vi "Curtin_convertrawData.vi"(0 "incoming data":waveform(dbl)[](array[waveform]), 1 "Ports":cluster{"mic":u8, "hammer":u8, "flip?":bool}={"mic"=1, "hammer"=2, "flip?"=FALSE}) -> (2 "Ordered":waveform(dbl)[](array[waveform]))   [LabVIEW 2022 SP3]
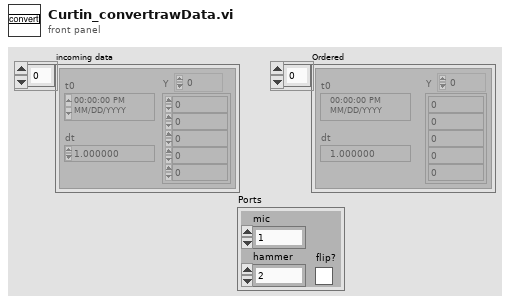
[diagram p1: front panel]
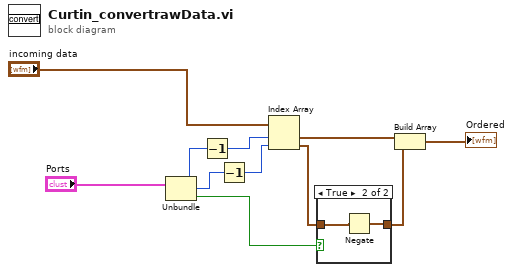
[diagram p0: block diagram]
diagram:
  n1 = Unbundle("Ports") -> ("mic"=w10:u8, "hammer"=w9:u8, "flip?"=w3:bool)
  n2 = Decrement(x=w10) -> (x-1=w2:u8)
  n3 = Decrement(x=w9) -> (x-1=w1:u8)
  n4 = Index Array(array="incoming data", index #1=w2, index #2=w1) -> (element #1=w8:waveform(dbl), element #2=w6:waveform(dbl))
  n5 = case shown="True" w3 {
    tunnel: w6 -> [w12 w14]
    tunnel: [w12 w13] -> w5
    frame False {
    }
    frame True {
      n6 = Negate(x=w14) -> (-x=w13:waveform(dbl))
    }
  }
  n7 = Build Array(w8, w5) -> (→"Ordered":waveform(dbl)[])
